vi "girpcutil_RpcValue_Get.vi"(0 "girpcutil_params":T1, 6 "Fehler (Eingang, kein Fehler)":errorcluster, 10 "member":string, 14 "value":i32) -> (20 "StringResult":string, 21 "Int64Result":i64, 22 "StructResult":i32, 25 "BoolResult":bool, 26 "Fehler (Ausgang)":errorcluster)   [LabVIEW 2016]
uses:
  girpcutil_params.ctl
panel:
  out "resultLen":i32
  out "errMsg 2":u8[](array[numeric])
  out "errMsgLen 2":i32
  out "type":u32
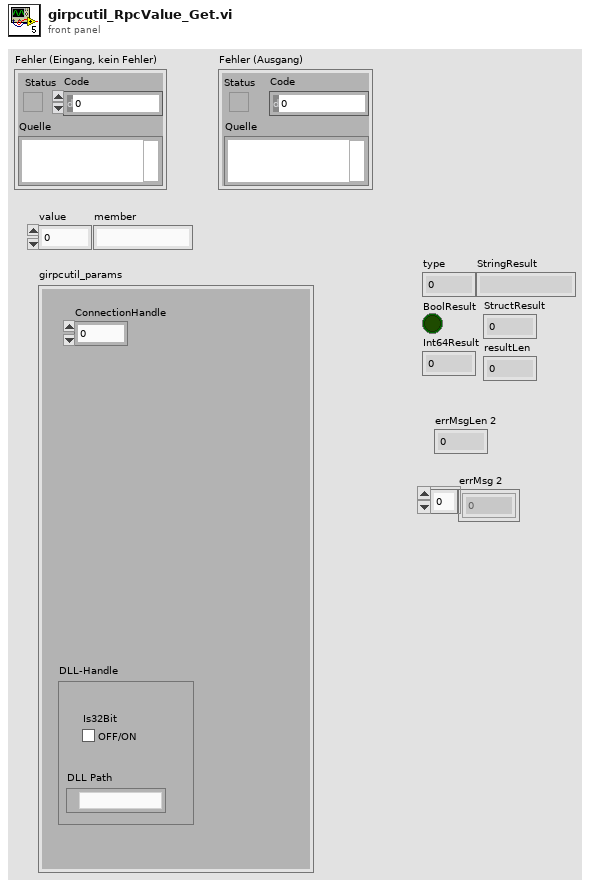
[diagram p1: front panel]
types:
  T1 = typedef "girpcutil_params.ctl" = cluster{"ConnectionHandle":i32, "DLL-Handle":cluster{"DLL Path":path, "Is32Bit":bool}}
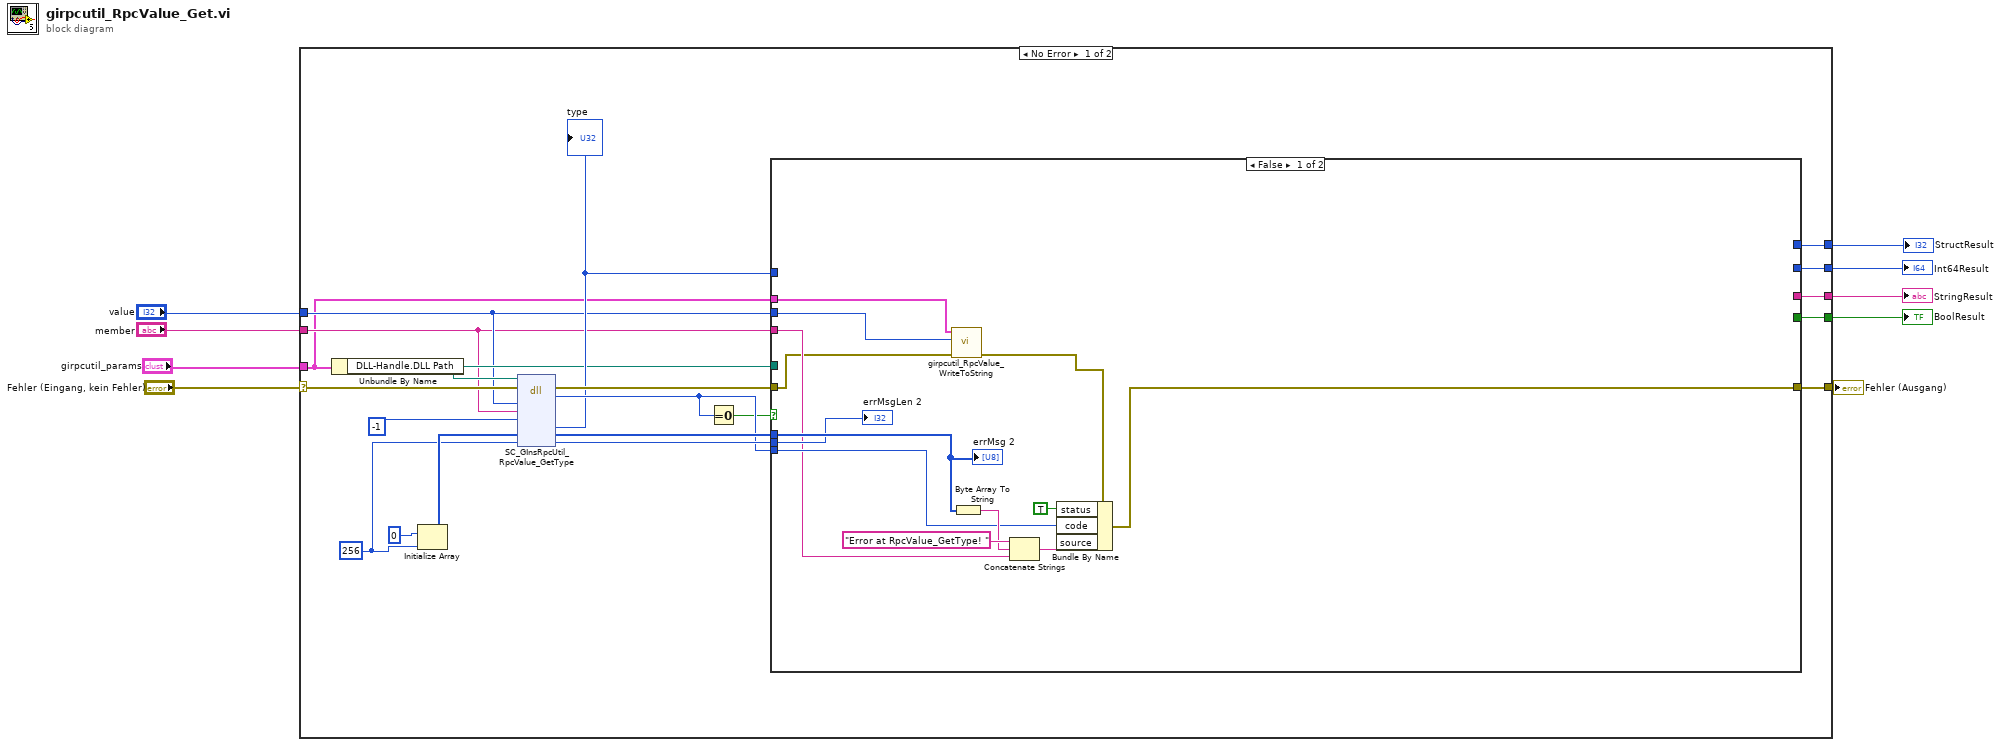
[diagram p0: block diagram]
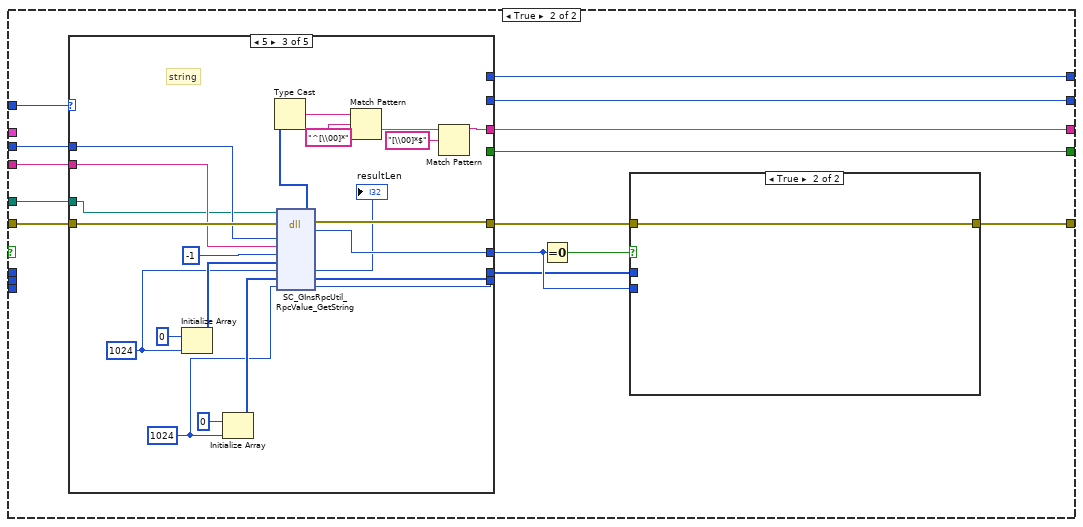
[diagram p2: hidden frame]
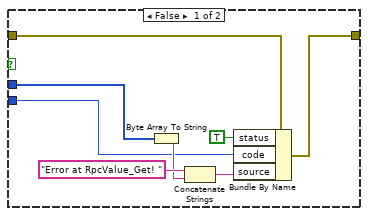
[diagram p3: hidden frame]
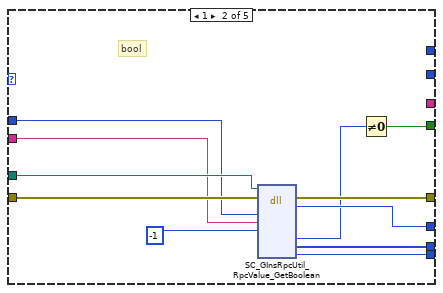
[diagram p5: hidden frame]
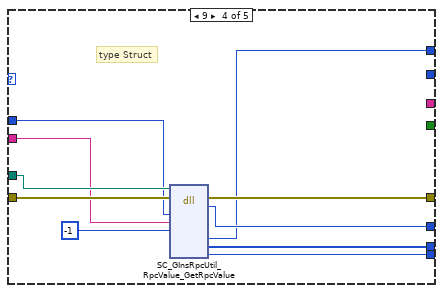
[diagram p6: hidden frame]
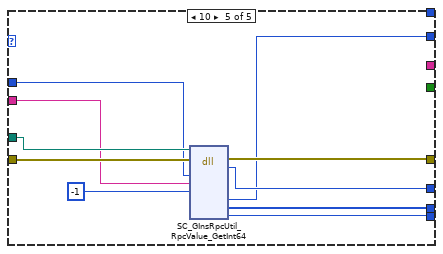
[diagram p7: hidden frame]
diagram:
  n1 = case shown="No Error" "Fehler (Eingang, kein Fehler)" {
    selector: "Fehler (Eingang, kein Fehler)" -> [w29 w120]
    tunnel: [w26 w120] -> w8
    tunnel: "girpcutil_params" -> [w13 _]
    tunnel: "value" -> [w19 _]
    tunnel: "member" -> [w18 _]
    tunnel: [w17 _] -> w4
    tunnel: [w16 _] -> w3
    tunnel: [w15 _] -> w2
    tunnel: [w14 _] -> w1
    frame No Error {
      w10 = 256 ("dimension size")
      n2 = Unbundle By Name(w13) -> ("DLL-Handle.DLL Path"=w20:path)
      n3 = Initialize Array(0, w10) -> (w11:i32[])
      n4 = dll-call lib="?" fn="SC_GInsRpcUtil_RpcValue_GetType"(path in=w20, error in=w29, "value"=w19, "member"=w18, "index"=-1, "errMsg"=w11, "errMsgLen"=w10) -> (error out=w27:errorcluster, "Rückgabewert"=w23:i32, "type"=w21:u32, "errMsg"=w24:u8[], "errMsgLen"=w25:i32)  [unwired: 5 in, 1 out]
      "type" <- w21
      n5 = Equal To 0?(x=w23) -> (x = 0?=w22:bool)
      n6 = case shown="False" w22 {
        tunnel: w27 -> [w33 w55]
        tunnel: [w36 w51] -> w26
        tunnel: w24 -> [w40 _]
        tunnel: w25 -> [w37 _]
        tunnel: w23 -> [w35 _]
        tunnel: w21 -> [_ w56]
        tunnel: w20 -> [_ w54]
        tunnel: w19 -> [w30 w53]
        tunnel: w18 -> [w34 w52]
        tunnel: [_ w46] -> w17
        tunnel: [_ w45] -> w16
        tunnel: [_ w44] -> w15
        tunnel: [_ w43] -> w14
        tunnel: w13 -> [w31 _]
        frame False {
          n7 = call "girpcutil_RpcValue_WriteToString.vi"("Fehler (Eingang, kein Fehler)"=w33, "value"=w30, "girpcutil_params"=w31) -> ("Fehler (Ausgang)"=w32:errorcluster)  [unwired: 8 in]
          n8 = Byte Array To String(unsigned byte array=w40) -> (string=w41:string)
          n9 = Concatenate Strings("Error at RpcValue_GetType! " ("source"), w41, w34) -> (w39:string)
          n10 = Bundle By Name(cluster=w32, "status"=TRUE, "code"=w35, "source"=w39) -> (w36:errorcluster)
          "errMsg 2" <- w40
          "errMsgLen 2" <- w37
        }
        frame True {
          n11 = case shown="5" w56 {
            tunnel: w55 -> [w66 w77 w99 w109 w119]
            tunnel: w54 -> [_ w76 w96 w107 w117]
            tunnel: w53 -> [_ w75 w98 w106 w116]
            tunnel: w52 -> [_ w74 w97 w105 w115]
            tunnel: [w66 w72 w92 w108 w118] -> w50
            tunnel: [_ w71 w93 w101 w111] -> w48
            tunnel: [_ w70 w95 w103 w113] -> w47
            tunnel: [_ w69 w94 w102 w112] -> _
            tunnel: [_ w67 _ _ _] -> w46
            tunnel: [_ _ w83 _ _] -> w45
            tunnel: [_ _ _ _ w110] -> w44
            tunnel: [_ _ _ w100 _] -> w43
            frame 0, Default {
            }
            frame 1 {
              # "bool"
              n12 = dll-call lib="?" fn="SC_GInsRpcUtil_RpcValue_GetBoolean"(path in=w76, error in=w77, "value"=w75, "member"=w74, "index"=-1) -> (error out=w72:errorcluster, "Rückgabewert"=w71:i32, "result"=w68:u8, "errMsg"=w70:u8[], "errMsgLen"=w69:i32)  [unwired: 7 in, 1 out]
              n13 = Not Equal To 0?(x=w68) -> (x != 0?=w67:bool)
            }
            frame 5 {
              w78 = 1024 ("dimension size")
              w88 = 1024 ("dimension size")
              # "string"
              n14 = Initialize Array(u8 0, w88) -> (w89:u8[])
              n15 = Initialize Array(u8 0, w78) -> (w79:u8[])
              n16 = dll-call lib="?" fn="SC_GInsRpcUtil_RpcValue_GetString"(path in=w96, error in=w99, "value"=w98, "member"=w97, "index"=-1, "result"=w89, "resultLen"=w88, "errMsg"=w79, "errMsgLen"=w78) -> (error out=w92:errorcluster, "Rückgabewert"=w93:i32, "result"=w86:u8[], "resultLen"=→"resultLen":i32, "errMsg"=w95:u8[], "errMsgLen"=w94:i32)  [unwired: 4 in, 1 out]
              n17 = Type Cast(x=w86) -> (*(type *) &x=w85:string)  [unwired: 1 in]
              n18 = Match Pattern(string=w85, regular expression="^[\\00]*") -> (after substring=w84:string)  [unwired: 1 in, 3 out]
              n19 = Match Pattern(string=w84, regular expression="[\\00]*$") -> (before substring=w83:string)  [unwired: 1 in, 3 out]
            }
            frame 9 {
              # "type Struct"
              n20 = dll-call lib="?" fn="SC_GInsRpcUtil_RpcValue_GetRpcValue"(path in=w107, error in=w109, "value"=w106, "member"=w105, "index"=-1 ("result")) -> (error out=w108:errorcluster, "Rückgabewert"=w101:i32, "result"=w100:i32, "errMsg"=w103:u8[], "errMsgLen"=w102:i32)  [unwired: 7 in, 1 out]
            }
            frame 10 {
              n21 = dll-call lib="?" fn="SC_GInsRpcUtil_RpcValue_GetInt64"(path in=w117, error in=w119, "value"=w116, "member"=w115, "index"=-1) -> (error out=w118:errorcluster, "Rückgabewert"=w111:i32, "result"=w110:i64, "errMsg"=w113:u8[], "errMsgLen"=w112:i32)  [unwired: 7 in, 1 out]
            }
          }
          n22 = Equal To 0?(x=w48) -> (x = 0?=w49:bool)
          n23 = case shown="True" w49 {
            tunnel: w50 -> [w59 w65]
            tunnel: [w58 w65] -> w51
            tunnel: w47 -> [w62 _]
            tunnel: w48 -> [w57 _]
            frame False {
              n24 = Byte Array To String(unsigned byte array=w62) -> (string=w63:string)
              n25 = Concatenate Strings("Error at RpcValue_Get! " ("source"), w63) -> (w61:string)
              n26 = Bundle By Name(cluster=w59, "status"=TRUE, "code"=w57, "source"=w61) -> (w58:errorcluster)
            }
            frame True {
            }
          }
        }
      }
    }
    frame Error {
    }
  }
  "Fehler (Ausgang)" <- w8
  "BoolResult" <- w4
  "StringResult" <- w3
  "Int64Result" <- w2
  "StructResult" <- w1
